vi "Periodic Tasks.vi"(8 "error in":errorcluster) -> ()   [LabVIEW 2014]
doc: "This VI runs in parallel to other tasks. It can contain as many user-defined periodic loops as you need. These can carry out PID or other sorts of timed response."
uses:
  <vilib>/Rock Robotics/WPI/DriverStation/WPI_DriverStationRobotMode2.ctl
  <vilib>/Rock Robotics/WPI/Joystick/WPI_JoystickGetSetRefNum.vi
  <vilib>/Rock Robotics/WPI/RobotDrive/WPI_RobotDriveGetSetRefNum.vi
  Global Variables.vi
  Robot Global Data.vi
  <vilib>/addons/control/pid/NI_PID_pid.lvlib
  <vilib>/addons/control/pid/pid.llb/PID (DBL).vi
panel:
  in  "PID gains":T1={"proportional gain (Kc)"=1.0, "integral time (Ti, min)"=0.01, "derivative time (Td, min)"=0.0} {"derivative time (Td, min)" format="%.3f"; "integral time (Ti, min)" format="%.3f"; "proportional gain (Kc)" format="%.3f"}
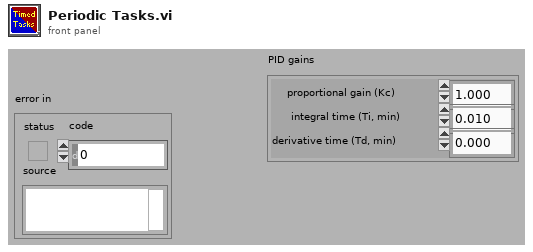
[diagram p1: front panel]
types:
  T1 = cluster{"proportional gain (Kc)":dbl, "integral time (Ti, min)":dbl, "derivative time (Td, min)":dbl}
  T2 = enum16{"Stop", "Three Tote", "Two Tote", "One Tote", "Step", "Top", "Home", "Joystick"}
  T3 = typedef "WPI_JoystickDevRef.ctl" = cluster{"Device":T4}
  T4 = typedef "WPI_JoystickDeviceEnum.ctl" = enum16{"USB 0", "USB 1", "USB 2", "USB 3", "USB 4", "USB 5"}
  T5 = typedef "WPI_RobotDriveDevRef.ctl" = cluster{"DevStatus":errorcluster, "Motors[]":T6[], "Square Inputs":bool, "Max Output":dbl}
  T6 = typedef "WPI_MotorControlDeviceRef.ctl" = cluster{"DeviceStatus":errorcluster, "Type":T7, "PWM":cluster{"Controller":T8, "PWM Channel":T9, "DeadBand":T10}, "CAN":cluster{"Device Number":u8, "Control Mode":T11, "Semaphore":T12, "Max Vout":dbl, "TalonSRX Control Mode":T13}, "Invert":bool, "TransformRef":T14, "InvTransformRef":T14}
  T7 = typedef "WPI_MotorControlType.ctl" = enum16{"PWM", "CAN", "CANTalonSRX"}
  T8 = typedef "FPGA_TypedefDigitalModule.ctl" = enum16{"Controller 1"}
  T9 = typedef "FPGA_DIOPWMChannel.ctl" = enum8{"PWM 0", "PWM 1", "PWM 2", "PWM 3", "PWM 4", "PWM 5", "PWM 6", "PWM 7", "PWM 8", "PWM 9", "PWM MXP 0", "PWM MXP 1", "PWM MXP 2", "PWM MXP 3", "PWM MXP 4", "PWM MXP 5", "PWM MXP 6", "PWM MXP 7", "PWM MXP 8", "PWM MXP 9", "Invalid"}
  T10 = typedef "WPI_PWMDeadband.ctl" = cluster{"Name":string, "maxPositivePwm":i32, "minPositivePwm":i32, "centerPwm":i32, "maxNegativePwm":i32, "minNegativePwm":i32, "angularRange":u16}
  T11 = typedef "WPI_CANJaguar_ControlMode.ctl" = enum8{"Percent VBus", "Current", "Speed", "Position", "Voltage"}
  T12 = typedef "Semaphore RefNum" = refnum<k1>
  T13 = typedef "WPI_CANTalonSRX_APIControlMode.ctl" = enum8{"Percent VBus", "Speed", "Position", "Slave", "Unchanged / Invalid"}
  T14 = typedef "WPI_PWMTransform_ConPane.ctl" = refnum<vi>
  T15 = typedef "WPI_DriverStationRobotMode2.ctl" = enum16{"Autonomous Disabled", "Autonomous Enabled", "Teleop Disabled", "Teleop Enabled", "Disconnected", "Finish", "Test Disabled", "Test Enabled", "Emergency Stopped"}
  T16 = cluster{"JoystickDevRef":T3, "RobotDriveDevRef":T5}
  T17 = typedef "WPI_CounterDevRef.ctl" = cluster{"DevStatus":errorcluster, "CntIndex":T18}
  T18 = typedef "FPGA_CounterCtrSystemIndex.ctl" = enum8{"Ctr 0", "Ctr 1", "Ctr 2", "Ctr 3", "Ctr 4", "Ctr 5", "Ctr 6", "Ctr 7", "Invalid"}
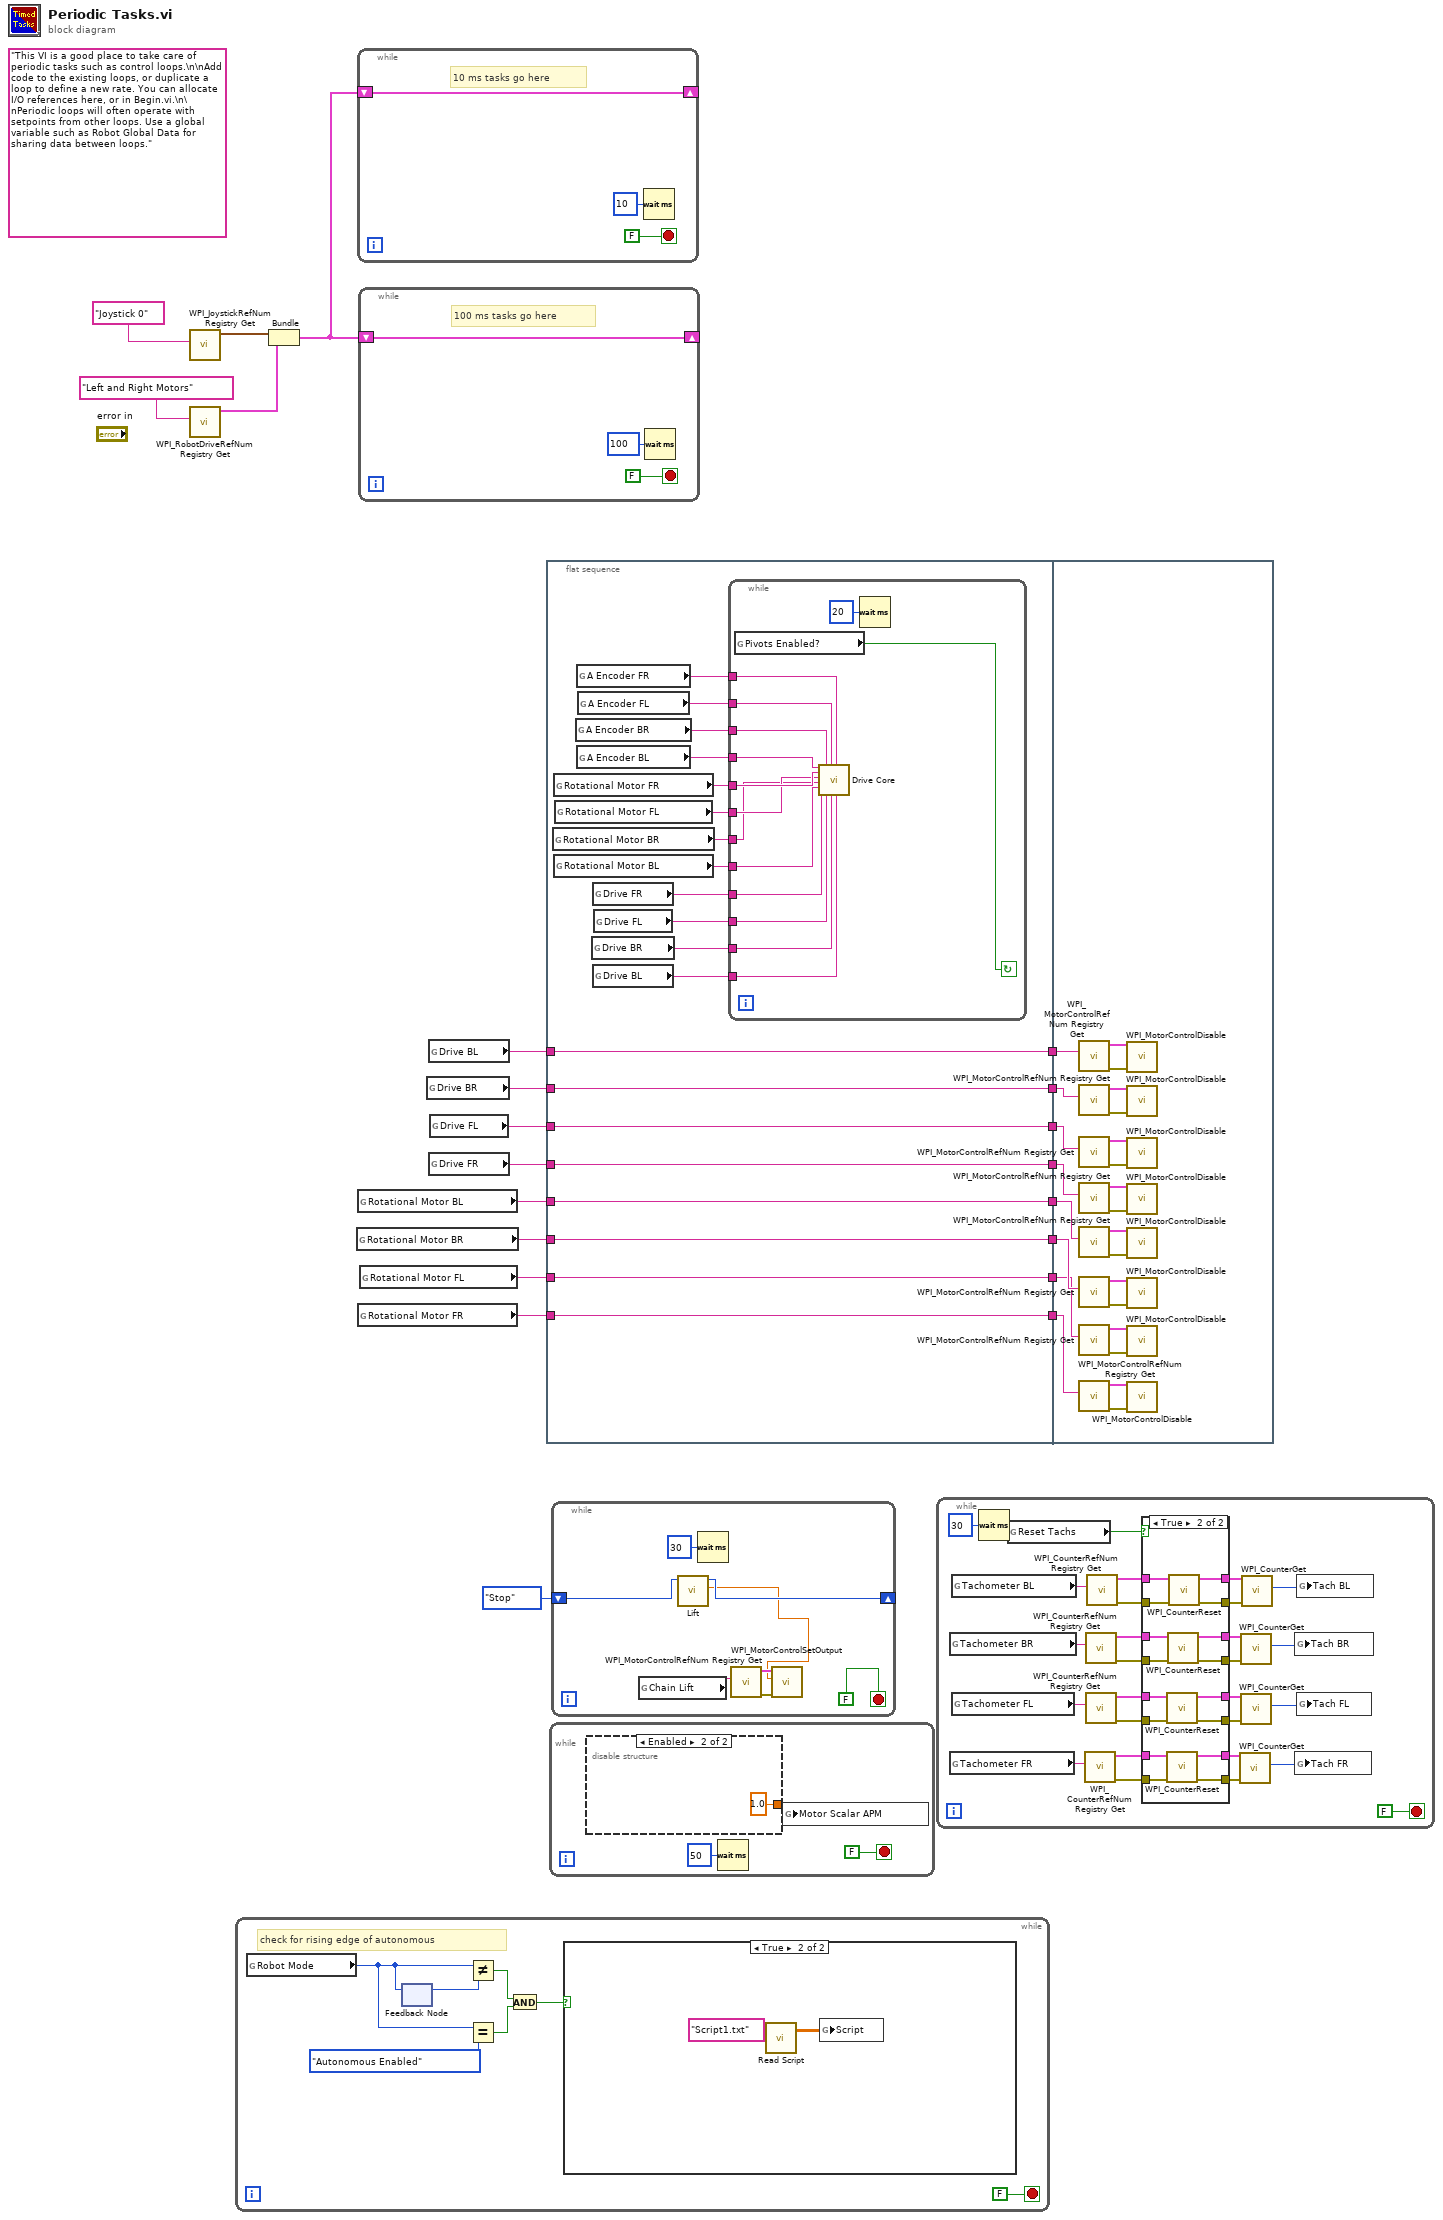
[diagram p0: block diagram]
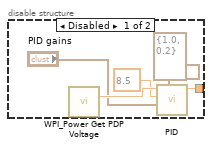
[diagram p4: hidden frame]
diagram:
  (unwired) "This VI is a good place to take care of periodic tasks such as control loops.\n\nAdd code to the existing loops, or duplicate a loop to define a new rate. You can allocate I/O references here, or in Begin.vi.\n\nPeriodic loops will often operate with setpoints from other loops. Use a global variable such as Robot Global Data for sharing data between loops."
  n1 = call <vilib>:"WPI_JoystickRefNum Registry Get.vi"("refnum name"="Joystick 0") -> ("JoystickDevRef"=w20:T3)  [unwired: 1 in, 9 out]
  n2 = call <vilib>:"WPI_RobotDriveRefNum Registry Get.vi"("refnum name"="Left and Right Motors") -> ("RobotDriveDevRef"=w19:T5)  [unwired: 1 in, 9 out]
  n3 = while {
    stop <- FALSE stop-if-true
    # "check for rising edge of autonomous"
    n4 = global read "Robot Global Data.vi" "Robot Mode"() -> (w27:T15)
    n5 = feedback #1() -> (w29:T15)  [unwired: 1 in]
    n6 = feedback-in #1(w27) -> ()
    n7 = Not Equal?(x=w27, y=w29) -> (x != y?=w25:bool)
    n8 = Equal?(x=w27, y=WPI_DriverStationRobotMode2."Autonomous Enabled" ("Robot Mode")) -> (x = y?=w26:bool)
    n9 = And(x=w25, y=w26) -> (x .and. y?=w23:bool)
    n10 = case shown="True" w23 {
      frame False {
      }
      frame True {
        n11 = call "Read Script.vi"("script name"="Script1.txt") -> ("output array"=w30:dbl[][])  [unwired: 1 in, 1 out]
        n12 = global write "Global Variables.vi" "Script"(w30) -> ()
      }
    }
  }
  n13 = Bundle("JoystickDevRef"=w20, "RobotDriveDevRef"=w19) -> (w18:T16)  [unwired: 1 out]
  n14 = global read "Global Variables.vi" "Rotational Motor BR"() -> (w6:string)
  n15 = while {
    shift-right: [w32] -> _
    shift-left: w18 -> [w32]
    stop <- FALSE stop-if-true
    # "10 ms tasks go here"
    n16 = Wait (ms)(milliseconds to wait=u32 10) -> ()  [unwired: 1 out]
  }
  n17 = global read "Global Variables.vi" "Rotational Motor BL"() -> (w8:string)
  n18 = global read "Global Variables.vi" "Rotational Motor FR"() -> (w2:string)
  n19 = while {
    shift-right: [w35] -> _
    shift-left: w18 -> [w35]
    stop <- FALSE stop-if-true
    # "100 ms tasks go here"
    n20 = Wait (ms)(milliseconds to wait=u32 100) -> ()  [unwired: 1 out]
  }
  n21 = global read "Global Variables.vi" "Rotational Motor FL"() -> (w4:string)
  n22 = global read "Global Variables.vi" "Drive BR"() -> (w14:string)
  n23 = global read "Global Variables.vi" "Drive BL"() -> (w16:string)
  n24 = global read "Global Variables.vi" "Drive FR"() -> (w10:string)
  n25 = global read "Global Variables.vi" "Drive FL"() -> (w12:string)
  n26 = flat-sequence {
    tunnel: [w45] -> w17
    tunnel: w16 -> [w45]
    tunnel: [w44] -> w15
    tunnel: w14 -> [w44]
    tunnel: [w43] -> w13
    tunnel: w12 -> [w43]
    tunnel: [w42] -> w11
    tunnel: w10 -> [w42]
    tunnel: [w41] -> w9
    tunnel: w8 -> [w41]
    tunnel: [w40] -> w7
    tunnel: w6 -> [w40]
    tunnel: [w39] -> w5
    tunnel: w4 -> [w39]
    tunnel: [w38] -> w3
    tunnel: w2 -> [w38]
    tunnel: w17 -> [w79]
    tunnel: w15 -> [w78]
    tunnel: w13 -> [w77]
    tunnel: w11 -> [w76]
    tunnel: w9 -> [w75]
    tunnel: w7 -> [w74]
    tunnel: w5 -> [w73]
    tunnel: w3 -> [w72]
    frame #0 {
      n27 = global read "Global Variables.vi" "Rotational Motor BR"() -> (w51:string)
      n28 = global read "Global Variables.vi" "Rotational Motor FR"() -> (w53:string)
      n29 = global read "Global Variables.vi" "Rotational Motor BL"() -> (w50:string)
      n30 = global read "Global Variables.vi" "Rotational Motor FL"() -> (w52:string)
      n31 = global read "Global Variables.vi" "A Encoder BR"() -> (w55:string)
      n32 = global read "Global Variables.vi" "A Encoder FR"() -> (w57:string)
      n33 = global read "Global Variables.vi" "A Encoder BL"() -> (w54:string)
      n34 = global read "Global Variables.vi" "A Encoder FL"() -> (w56:string)
      n35 = global read "Global Variables.vi" "Drive BR"() -> (w47:string)
      n36 = global read "Global Variables.vi" "Drive FR"() -> (w49:string)
      n37 = global read "Global Variables.vi" "Drive BL"() -> (w46:string)
      n38 = global read "Global Variables.vi" "Drive FL"() -> (w48:string)
      n39 = while {
        tunnel: w57 -> [w70]
        tunnel: w56 -> [w69]
        tunnel: w55 -> [w68]
        tunnel: w54 -> [w67]
        tunnel: w53 -> [w66]
        tunnel: w52 -> [w65]
        tunnel: w51 -> [w64]
        tunnel: w50 -> [w63]
        tunnel: w49 -> [w62]
        tunnel: w48 -> [w61]
        tunnel: w47 -> [w60]
        tunnel: w46 -> [w59]
        stop <- w71 continue-if-true
        n40 = global read "Global Variables.vi" "Pivots Enabled?"() -> (w71:bool)
        n41 = call "Drive Core.vi"("A Encoder BL"=w67, "Rotational Motor FR"=w66, "Rotational Motor FL"=w65, "Rotational Motor BR"=w64, "Rotational Motor BL"=w63, "Drive Motor FR"=w62, "A Encoder BR"=w68, "Drive Motor FL"=w61, "A Encoder FL"=w69, "Drive Motor BR"=w60, "A Encoder FR"=w70, "Drive Motor BL"=w59) -> ()  [unwired: 8 in]
        n42 = Wait (ms)(milliseconds to wait=u32 20) -> ()  [unwired: 1 out]
      }
    }
    frame #1 {
      n43 = call <vilib>:"WPI_MotorControlRefNum Registry Get.vi"("refnum name"=w79) -> ("error out"=w95:errorcluster, "MotorControlDevRef"=w94:T6)  [unwired: 9 in]
      n44 = call <vilib>:"WPI_MotorControlRefNum Registry Get.vi"("refnum name"=w78) -> ("error out"=w93:errorcluster, "MotorControlDevRef"=w92:T6)  [unwired: 9 in]
      n45 = call <vilib>:"WPI_MotorControlRefNum Registry Get.vi"("refnum name"=w77) -> ("error out"=w91:errorcluster, "MotorControlDevRef"=w90:T6)  [unwired: 9 in]
      n46 = call <vilib>:"WPI_MotorControlRefNum Registry Get.vi"("refnum name"=w76) -> ("error out"=w89:errorcluster, "MotorControlDevRef"=w88:T6)  [unwired: 9 in]
      n47 = call <vilib>:"WPI_MotorControlRefNum Registry Get.vi"("refnum name"=w75) -> ("error out"=w87:errorcluster, "MotorControlDevRef"=w86:T6)  [unwired: 9 in]
      n48 = call <vilib>:"WPI_MotorControlRefNum Registry Get.vi"("refnum name"=w74) -> ("error out"=w85:errorcluster, "MotorControlDevRef"=w84:T6)  [unwired: 9 in]
      n49 = call <vilib>:"WPI_MotorControlRefNum Registry Get.vi"("refnum name"=w73) -> ("error out"=w83:errorcluster, "MotorControlDevRef"=w82:T6)  [unwired: 9 in]
      n50 = call <vilib>:"WPI_MotorControlRefNum Registry Get.vi"("refnum name"=w72) -> ("error out"=w81:errorcluster, "MotorControlDevRef"=w80:T6)  [unwired: 9 in]
      n51 = call <vilib>:"WPI_MotorControlDisable.vi"("error in (no error)"=w95, "MotorControlDevRef"=w94) -> ()  [unwired: 8 in, 2 out]
      n52 = call <vilib>:"WPI_MotorControlDisable.vi"("error in (no error)"=w93, "MotorControlDevRef"=w92) -> ()  [unwired: 8 in, 2 out]
      n53 = call <vilib>:"WPI_MotorControlDisable.vi"("error in (no error)"=w91, "MotorControlDevRef"=w90) -> ()  [unwired: 8 in, 2 out]
      n54 = call <vilib>:"WPI_MotorControlDisable.vi"("error in (no error)"=w89, "MotorControlDevRef"=w88) -> ()  [unwired: 8 in, 2 out]
      n55 = call <vilib>:"WPI_MotorControlDisable.vi"("error in (no error)"=w87, "MotorControlDevRef"=w86) -> ()  [unwired: 8 in, 2 out]
      n56 = call <vilib>:"WPI_MotorControlDisable.vi"("error in (no error)"=w85, "MotorControlDevRef"=w84) -> ()  [unwired: 8 in, 2 out]
      n57 = call <vilib>:"WPI_MotorControlDisable.vi"("error in (no error)"=w83, "MotorControlDevRef"=w82) -> ()  [unwired: 8 in, 2 out]
      n58 = call <vilib>:"WPI_MotorControlDisable.vi"("error in (no error)"=w81, "MotorControlDevRef"=w80) -> ()  [unwired: 8 in, 2 out]
    }
  }
  n59 = while {
    stop <- FALSE stop-if-true
    n60 = disable-structure shown="Enabled" {
      disable-tunnel: [w99 1.0 ("Motor Scalar APM")] -> w96
      frame Disabled {
        n61 = call <vilib>:"WPI_Power Get PDP Voltage.vi"() -> ("voltage (V)"=w102:dbl)  [unwired: 14 in, 1 out]
        n62 = call-poly <vilib>:"PID.vi"("output range"=cluster{"output high":dbl, "output low":dbl} {"output high"=1.0, "output low"=0.2}, "PID gains"="PID gains", "process variable"=8.5 ("setpoint"), "setpoint"=w102) -> ("output"=w99:dbl)  [unwired: 6 in, 1 out]
      }
      frame Enabled {
      }
    }
    n63 = Wait (ms)(milliseconds to wait=u32 50) -> ()  [unwired: 1 out]
    n64 = global write "Global Variables.vi" "Motor Scalar APM"(w96) -> ()
  }
  n65 = while {
    shift-right: [w110] -> _
    shift-left: T2."Stop" ("State Out") -> [w111]
    stop <- FALSE stop-if-true
    n66 = global read "Global Variables.vi" "Chain Lift"() -> (w105:string)
    n67 = call "Lift.vi"("State"=w111) -> ("Lift Motor(Global...)"=w106:dbl, "State Out"=w110:T2)  [unwired: 9 in]
    n68 = Wait (ms)(milliseconds to wait=u32 30) -> ()  [unwired: 1 out]
    n69 = call <vilib>:"WPI_MotorControlRefNum Registry Get.vi"("refnum name"=w105) -> ("error out"=w109:errorcluster, "MotorControlDevRef"=w108:T6)  [unwired: 9 in]
    n70 = call <vilib>:"WPI_MotorControlSetOutput.vi"("error in (no error)"=w109, "Output"=w106, "MotorControlDevRef"=w108) -> ()  [unwired: 6 in, 3 out]
  }
  n71 = while {
    stop <- FALSE stop-if-true
    n72 = global read "Global Variables.vi" "Tachometer BR"() -> (w126:string)
    n73 = global read "Global Variables.vi" "Tachometer FR"() -> (w114:string)
    n74 = global read "Global Variables.vi" "Tachometer BL"() -> (w138:string)
    n75 = global read "Global Variables.vi" "Tachometer FL"() -> (w125:string)
    n76 = Wait (ms)(milliseconds to wait=u32 30) -> ()  [unwired: 1 out]
    n77 = global read "Global Variables.vi" "Reset Tachs"() -> (w137:bool)
    n78 = call <vilib>:"WPI_CounterRefNum Registry Get.vi"("refnum name"=w114) -> ("error out"=w116:errorcluster, "CounterDevRef"=w115:T17)  [unwired: 9 in]
    n79 = call <vilib>:"WPI_CounterRefNum Registry Get.vi"("refnum name"=w126) -> ("error out"=w128:errorcluster, "CounterDevRef"=w127:T17)  [unwired: 9 in]
    n80 = call <vilib>:"WPI_CounterRefNum Registry Get.vi"("refnum name"=w125) -> ("error out"=w123:errorcluster, "CounterDevRef"=w124:T17)  [unwired: 9 in]
    n81 = call <vilib>:"WPI_CounterRefNum Registry Get.vi"("refnum name"=w138) -> ("error out"=w135:errorcluster, "CounterDevRef"=w136:T17)  [unwired: 9 in]
    n82 = case shown="True" w137 {
      tunnel: w136 -> [w147 w163]
      tunnel: w135 -> [w146 w162]
      tunnel: [w147 w161] -> w134
      tunnel: [w146 w160] -> w133
      tunnel: w127 -> [w144 w150]
      tunnel: w128 -> [w145 w159]
      tunnel: [w144 w149] -> w129
      tunnel: [w145 w148] -> w130
      tunnel: w124 -> [w143 w151]
      tunnel: w123 -> [w142 w158]
      tunnel: [w143 w152] -> w122
      tunnel: [w142 w153] -> w121
      tunnel: w115 -> [w140 w156]
      tunnel: w116 -> [w141 w157]
      tunnel: [w140 w155] -> w117
      tunnel: [w141 w154] -> w118
      frame False {
      }
      frame True {
        n83 = call <vilib>:"WPI_CounterReset.vi"("error in (no error)"=w158, "CounterDevRef in"=w151) -> ("error out"=w153:errorcluster, "CounterDevRef out"=w152:T17)  [unwired: 8 in]
        n84 = call <vilib>:"WPI_CounterReset.vi"("error in (no error)"=w157, "CounterDevRef in"=w156) -> ("error out"=w154:errorcluster, "CounterDevRef out"=w155:T17)  [unwired: 8 in]
        n85 = call <vilib>:"WPI_CounterReset.vi"("error in (no error)"=w159, "CounterDevRef in"=w150) -> ("error out"=w148:errorcluster, "CounterDevRef out"=w149:T17)  [unwired: 8 in]
        n86 = call <vilib>:"WPI_CounterReset.vi"("error in (no error)"=w162, "CounterDevRef in"=w163) -> ("error out"=w160:errorcluster, "CounterDevRef out"=w161:T17)  [unwired: 8 in]
      }
    }
    n87 = call <vilib>:"WPI_CounterGet.vi"("error in (no error)"=w118, "CounterDevRef in"=w117) -> ("Value"=w119:i32)  [unwired: 4 in, 5 out]
    n88 = call <vilib>:"WPI_CounterGet.vi"("error in (no error)"=w130, "CounterDevRef in"=w129) -> ("Value"=w131:i32)  [unwired: 4 in, 5 out]
    n89 = call <vilib>:"WPI_CounterGet.vi"("error in (no error)"=w121, "CounterDevRef in"=w122) -> ("Value"=w120:i32)  [unwired: 4 in, 5 out]
    n90 = call <vilib>:"WPI_CounterGet.vi"("error in (no error)"=w133, "CounterDevRef in"=w134) -> ("Value"=w132:i32)  [unwired: 4 in, 5 out]
    n91 = global write "Global Variables.vi" "Tach BR"(w131) -> ()
    n92 = global write "Global Variables.vi" "Tach FR"(w119) -> ()
    n93 = global write "Global Variables.vi" "Tach BL"(w132) -> ()
    n94 = global write "Global Variables.vi" "Tach FL"(w120) -> ()
  }
